vi "Evaluate.vi"(0 "object in":refnum<class "OutOfGoalieArea.lvclass">, 1 "Game":refnum<class "Game.lvclass">, 2 "Point":dbl[](array[numeric]), 3 "Ally?":bool, 5 "error in (no error)":errorcluster) -> (14 "object out":refnum<class "OutOfGoalieArea.lvclass">, 16 "Evaluation":dbl, 19 "error out":errorcluster)   [LabVIEW 2023, in "OutOfGoalieArea.lvclass"]
uses:
  OutOfGoalieArea.lvclass
  OutOfGoalieArea.lvclass/OutOfGoalieArea.ctl
  Field_class/Field.lvclass
  Game_class/Game.lvclass
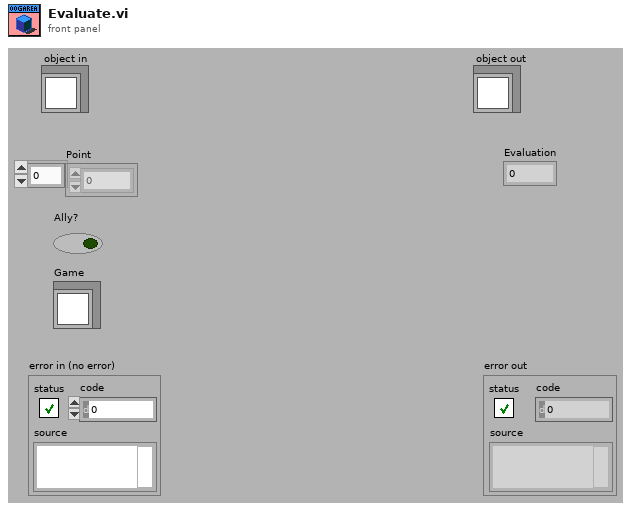
[diagram p1: front panel]
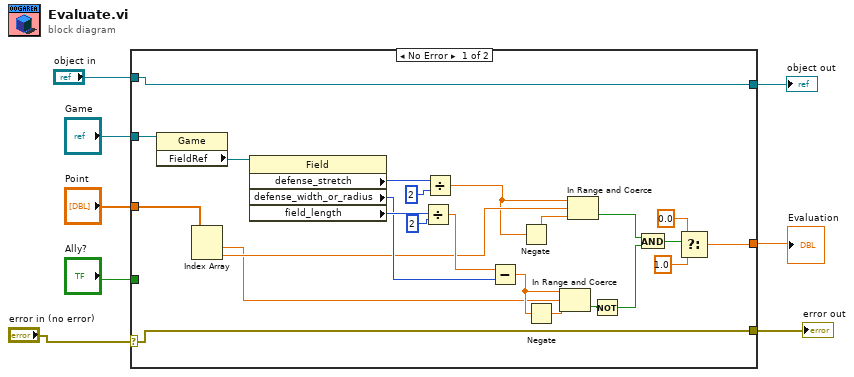
[diagram p0: block diagram]
diagram:
  n1 = case shown="No Error" "error in (no error)" {
    selector: "error in (no error)" -> [w32 w34]
    tunnel: [w32 w34] -> w7
    tunnel: "Game" -> [w31 _]
    tunnel: "Ally?" -> [_ _]
    tunnel: "Point" -> [w19 _]
    tunnel: [w13 _] -> w3
    tunnel: "object in" -> [w12 w33]
    tunnel: [w12 w33] -> w1
    frame No Error {
      n2 = property class="Game"(reference=w31) -> ("FieldRef"=w30:refnum<class "Field.lvclass">)  [unwired: 1 in, 2 out]
      n3 = Index Array(array=w19) -> (element #1=w17:dbl, element #2=w18:dbl)  [unwired: 2 in]
      n4 = property class="Field"(reference=w30) -> ("defense_stretch"=w11:i32, "defense_width_or_radius"=w25:i32, "field_length"=w28:i32)  [unwired: 1 in, 2 out]
      n5 = Divide(x=w28, y=2) -> (x/y=w26:dbl)
      n6 = Divide(x=w11, y=2) -> (x/y=w10:dbl)
      n7 = Subtract(x=w26, y=w25) -> (x-y=w23:dbl)
      n8 = Negate(x=w10) -> (-x=w29:dbl)
      n9 = Negate(x=w23) -> (-x=w24:dbl)
      n10 = In Range and Coerce(upper limit=w23, x=w17, lower limit=w24) -> (In Range?=w22:bool)  [unwired: 1 out]
      n11 = In Range and Coerce(upper limit=w10, x=w18, lower limit=w29) -> (In Range?=w20:bool)  [unwired: 1 out]
      n12 = Not(x=w22) -> (.not. x?=w21:bool)
      n13 = And(x=w20, y=w21) -> (x .and. y?=w16:bool)
      n14 = Select(t=0.0, s=w16, f=1.0) -> (s? t:f=w13:dbl)
    }
    frame Error {
    }
  }
  "error out" <- w7
  "object out" <- w1
  "Evaluation" <- w3
